vi "Set Debug Flag.vi"(8 "error in (no error)":errorcluster, 10 "NewVal":bool, 11 "Active Project":path) -> (0 "error out":errorcluster)   [LabVIEW 2020, in "Main.lvclass"]
uses:
  Main.lvclass
  Conditional Disabled Configurator/Conditional Disabled Configurator.lvclass
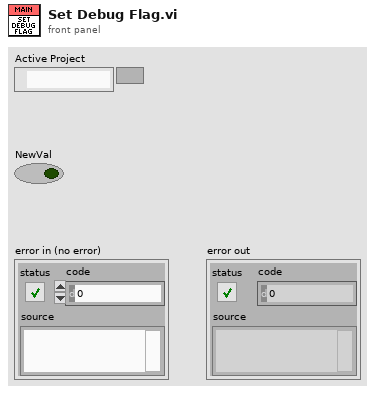
[diagram p1: front panel]
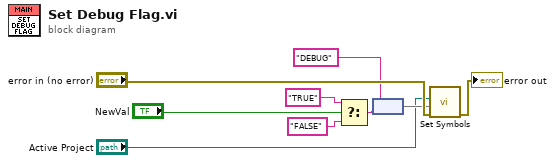
[diagram p0: block diagram]
diagram:
  n1 = Select(t="TRUE", s="NewVal", f="FALSE") -> (s? t:f=w5:string)
  n2 = node("DEBUG" ("key"), w5) -> (w6:map{string, string})
  n3 = call "Set Symbols.vi"("error in (no error)"="error in (no error)", "Symbols"=w6, "Project Path"="Active Project") -> ("error out"=→"error out":errorcluster)  [unwired: 8 in]
